vi "Detect Objects with YOLOV3-tiny.vi"() -> ()   [LabVIEW 2020, in "examples.lvlib"]
uses:
  examples.lvlib
  feature_detection/DNN Detection Model/Detection.ctl
  feature_detection/DNN Detection Model/Rectangle Corners.ctl
  common/Image Point (Integer).ctl
  feature_detection/DNN Detection Model/Model Parameters.ctl
  common/Image Size (Integer).ctl
  common/Object Point (Float).ctl
  <vilib>/Utility/sysdir.llb/System Directory Type.ctl
  feature_detection/DNN Detection Model/DNN Detection Model.lvclass/DNN Detection Model.ctl
  image/ARGB Colour.ctl
  image/New Image (ARGB Preallocated).vi
  image/Copy Pixmap to Image (ARGB Flatten Mask).vi
  feature_detection/DNN Detection Model/Detect (ARGB).vi
  image/Draw Rectangle (ARGB).vi
  image/Draw Text (ARGB).vi
  image/Draw Image to Picture (ARGB).vi
  image/New Image (ARGB Preallocated).vi/3321fa97-f432-4e1e-8db9-a0df79aed21b.vi
  image/ARGB Colour to U32 Pixel Value.vi
  image/Copy Pixmap to Image (ARGB Flatten Mask).vi/7d03ccf7-b889-4e8d-9f2a-57831e73dbde.vi
  feature_detection/DNN Detection Model/Detect (ARGB).vi/e837249a-f575-44a9-ab73-66ed6d7d79a4.vi
  image/Draw Rectangle (ARGB).vi/7e6fb015-3761-4366-a0a7-e436eb229083.vi
  image/Draw Text (ARGB).vi/0015c4fc-6a12-4f82-815b-6c2f827f408b.vi
  image/Draw Image to Picture (ARGB).vi/8cd07b1b-062e-4fe4-9e87-2eb3dc89fe0e.vi
  image/FixPixmap.vi
  image/Default8bitColourMap.vi
  <vilib>/Utility/file.llb/Read Delimited Spreadsheet (string).vi
  feature_detection/DNN Detection Model/Create (Darknet).vi
  <vilib>/Utility/error.llb/Error Cluster From Error Code.vi
  feature_detection/DNN Detection Model/DNN Detection Model.lvclass
  common/common.lvlib
  image/image.lvlib
  <vilib>/picture/picture.llb/imagedata.ctl
panel:
  out "Picture":picture
  out "Detections":T1[](array[typedef])
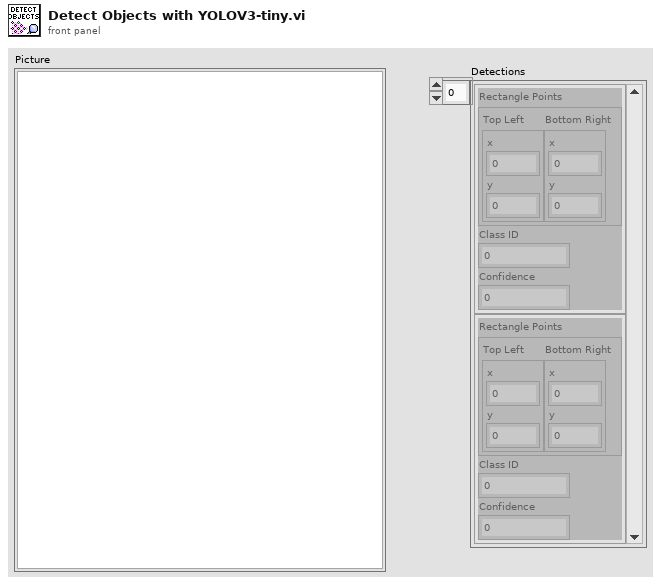
[diagram p1: front panel]
types:
  T1 = typedef "feature_detection.lvlib/DNN Detection Model.lvclass/Detection.ctl" = cluster{"Rectangle Points":T2, "Class ID":i32, "Confidence":sgl}
  T2 = typedef "feature_detection.lvlib/DNN Detection Model.lvclass/Rectangle Corners.ctl" = cluster{"Top Left":T3, "Bottom Right":T3}
  T3 = typedef "common.lvlib/Image Point (Integer).ctl" = cluster{"x":i32, "y":i32}
  T4 = typedef "feature_detection.lvlib/DNN Detection Model.lvclass/Model Parameters.ctl" = cluster{"Image Size":T5, "Mean":T6, "Scale":dbl, "Expects RGB Channel Order":bool, "Crop":bool}
  T5 = typedef "common.lvlib/Image Size (Integer).ctl" = cluster{"Width":u16, "Height":u16}
  T6 = typedef "common.lvlib/Object Point (Float).ctl" = cluster{"x":dbl, "y":dbl, "z":dbl}
  T7 = typedef "System Directory Type.ctl" = i32
  T8 = typedef "imagedata.ctl" = cluster{"image type":i32, "image depth":i32, "image":u8[], "mask":u8[], "colors":u32[], "Rectangle":cluster{"left":i16, "top":i16, "right":i16, "bottom":i16}}
  T9 = typedef "image.lvlib/ARGB Image.ctl" = refnum<data-value>
  T10 = typedef "image.lvlib/ARGB Colour.ctl" = cluster{"Alpha":u8, "RGB":u32}
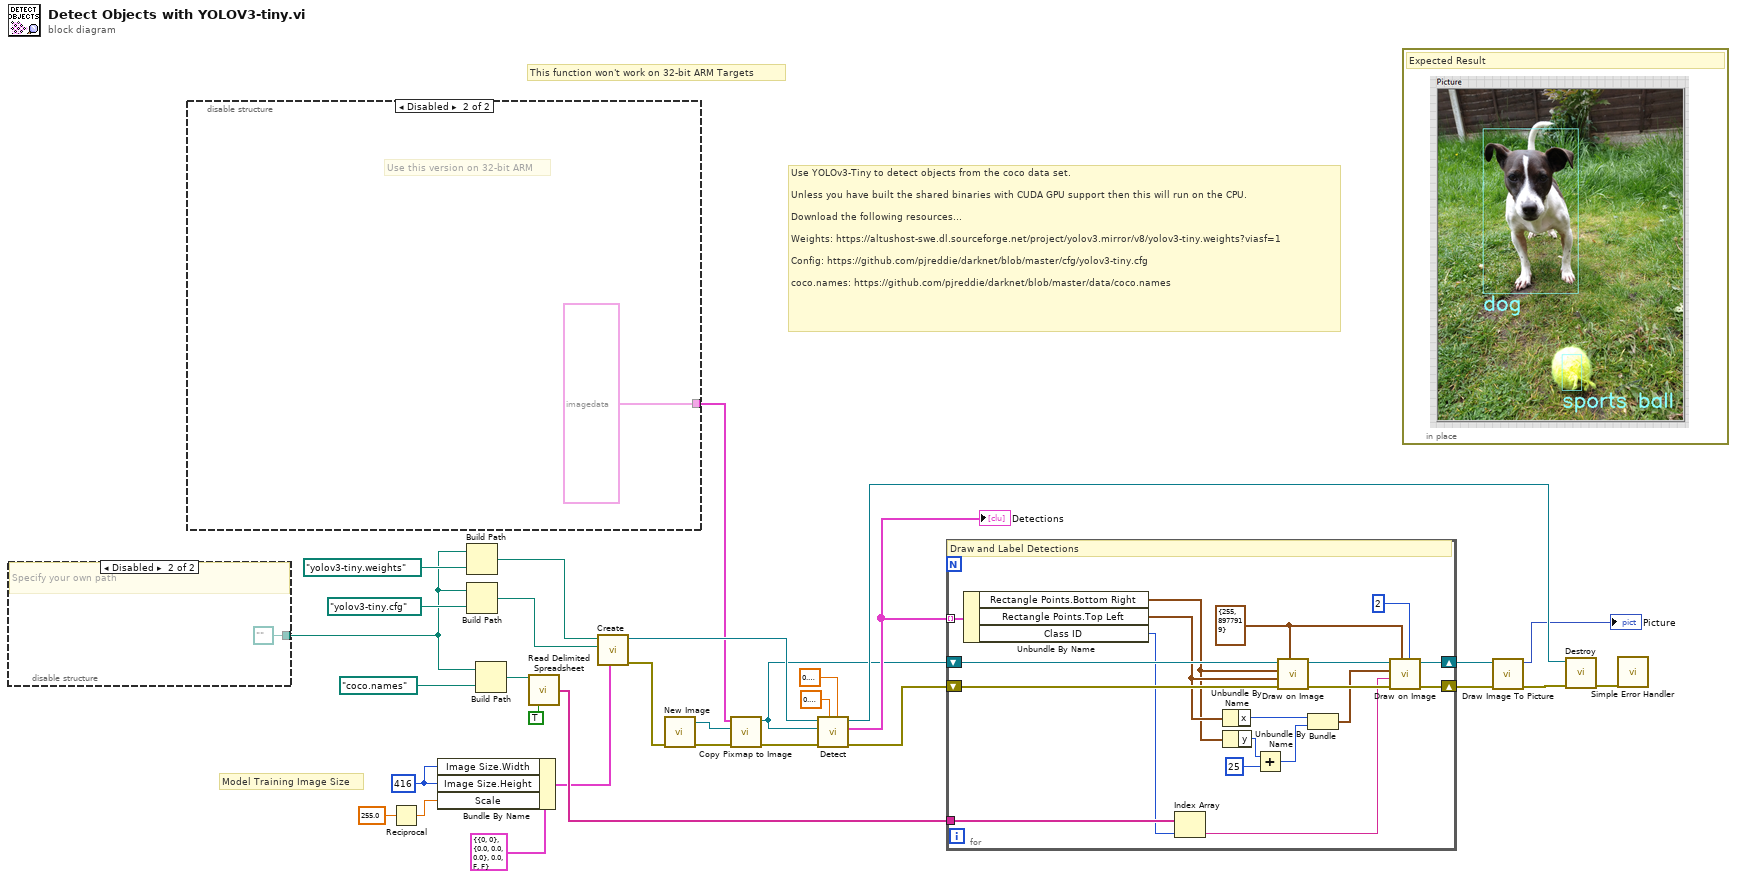
[diagram p0: block diagram]
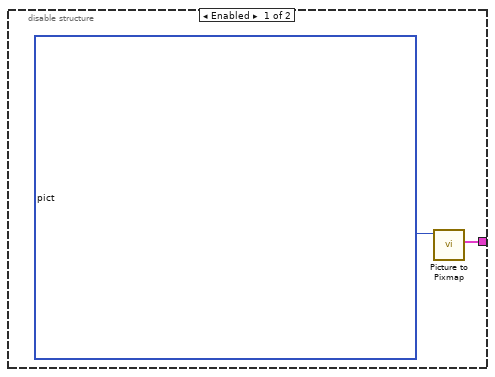
[diagram p2: hidden frame]
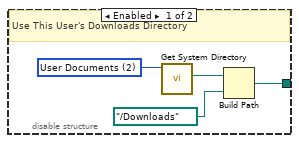
[diagram p3: hidden frame]
diagram:
  w19 = u16 416 ("Image Size.Width")
  # "This function won't work on 32-bit ARM Targets"
  # "Model Training Image Size"
  # "Use YOLOv3-Tiny to detect objects from the coco data set.\n\nUnless you have built the shared binaries with CUDA GPU support then this will run on the CPU.\n\nDownload the following resources...\n\nWeights: https://altushost-swe.dl.sourceforge.net/project/yolov3.mirror/v8/yolov3-tiny.weights?viasf=1\n\nConfig: https://github.com/pjreddie/darknet/blob/master/cfg/yolov3-tiny.cfg\n\ncoco.names: https://github.com/pjreddie/darknet/blob/master/data/coco.names"
  n1 = disable-structure shown="Disabled" {
    disable-tunnel: [w32 path "" ("appended path")] -> w16
    frame Enabled {
      w35 = T7 2 items=["User Home"=0, "User Desktop"=1, "User Documents"=2, "User Application Data"=3, "User Preferences"=4, "User Temporary"=5, "Public Documents"=6, "Public Application Data"=7, "Public Preferences"=8, "Public Cache"=13, "System Core Libraries"=9, "System Installed Libraries"=10, "Application Files"=11, "Boot Volume Root"=12] ("system directory type")
      # "Use This User's Downloads Directory"
      n2 = call <vilib>:"Get System Directory.vi"("system directory type"=w35) -> ("system directory"=w34:path)  [unwired: 10 in]
      n3 = Build Path(base path=w34, name or relative path=path "../Downloads") -> (appended path=w32:path)
    }
    frame Disabled {
      # "Specify your own path"
    }
  }
  n4 = disable-structure shown="Disabled" {
    disable-tunnel: [w37 T8 {"image type"=0, "image depth"=24, "image"=array[562500 elements], "mask"=[], "colors"=[], "Rectangle"={"left"=0, "top"=0, "right"=375, "bottom"=500}} ("image data")] -> w6
    frame Enabled {
      n5 = call <vilib>:"Picture to Pixmap.vi"("picture"=picture bytes[562530] ("Picture")) -> ("image data"=w37:T8)  [unwired: 9 in, 1 out]
    }
    frame Disabled {
      # "Use this version on 32-bit ARM"
    }
  }
  n6 = Reciprocal(x=255.0) -> (1/x=w20:dbl)
  n7 = Bundle By Name(cluster=T4 {"Image Size"={"Width"=0, "Height"=0}, "Mean"={"x"=0.0, "y"=0.0, "z"=0.0}, "Scale"=0.0, "Expects RGB Channel Order"=FALSE, "Crop"=FALSE} ("Image Handling Properties"), "Image Size.Width"=w19, "Image Size.Height"=w19, "Scale"=w20) -> (w21:T4)
  n8 = Build Path(base path=w16, name or relative path=path "yolov3-tiny.weights") -> (appended path=w26:path)
  n9 = Build Path(base path=w16, name or relative path=path "yolov3-tiny.cfg") -> (appended path=w23:path)
  n10 = Build Path(base path=w16, name or relative path=path "coco.names") -> (appended path=w13:path)
  n11 = call-poly <vilib>:"Read Delimited Spreadsheet.vi"("file path (dialog if empty)"=w13, "transpose? (F)"=TRUE) -> ("first row"=w31:string[])  [unwired: 8 in, 5 out]
  n12 = call-poly "Create.vi"("Image Handling Properties"=w21, "Config (*.cfg)"=w23, "Darknet Weights (*.weights)"=w26) -> ("error out"=w30:errorcluster, "DNN Detection Model"=w28:refnum<class "DNN Detection Model.lvclass">)  [unwired: 7 in]
  n13 = call-poly "New Image.vi"("error in (no error)"=w30) -> ("error out"=w2:errorcluster, "ARGB Image"=w1:T9)  [unwired: 9 in]
  n14 = call-poly "Copy Pixmap to Image.vi"("error in (no error)"=w2, "ARGB Image Destination in"=w1, "Pixmap Image Data"=w6) -> ("error out"=w4:errorcluster, "ARGB Image Destination"=w3:T9)  [unwired: 7 in]
  n15 = call-poly "Detect.vi"("Non-Maxium Suppression Threshold"=sgl 0.1, "Confidence Threshold"=sgl 0.2, "error in (no error)"=w4, "ARGB Image in"=w3, "DNN Detection Model in"=w28) -> ("error out"=w12:errorcluster, "Detections"=w11:T1[], "DNN Detection Model"=w29:refnum<class "DNN Detection Model.lvclass">)  [unwired: 4 in]
  "Detections" <- w11
  n16 = for {
    tunnel: w11 -> [w58] mode=indexing
    shift-right: [w53] -> w9
    shift-left: w12 -> [w57]
    shift-right: [w52] -> w10
    shift-left: w3 -> [w56]
    tunnel: w31 -> [w55]
    w50 = T10 {"Alpha"=255, "RGB"=8977919} ("ARGB Colour")
    # "Draw and Label Detections"
    n17 = Unbundle By Name(w58) -> ("Rectangle Points.Bottom Right"=w45:T3, "Rectangle Points.Top Left"=w46:T3, "Class ID"=w47:i32)
    n18 = Index Array(array=w55, index=w47) -> (element=w49:string)
    n19 = Unbundle By Name(w46) -> ("x"=w44:i32)
    n20 = Unbundle By Name(w45) -> ("y"=w43:i32)
    n21 = Add(x=w43, y=25) -> (x+y=w41:i32)
    n22 = call-poly "Draw on Image.vi"("ARGB Colour"=w50, "error in (no error)"=w57, "Point B"=w46, "Point A"=w45, "ARGB Image in"=w56) -> ("error out"=w54:errorcluster, "ARGB Image"=w51:T9)  [unwired: 5 in]
    n23 = Bundle("x"=w44, w41) -> (w42:cluster{"x":i32, i32})  [unwired: 1 in]
    n24 = call-poly "Draw on Image.vi"("Thickness (Default: 1)"=2, "ARGB Colour"=w50, "error in (no error)"=w54, "Text"=w49, "Origin"=w42, "ARGB Image in"=w51) -> ("error out"=w53:errorcluster, "ARGB Image"=w52:T9)  [unwired: 4 in]
  }
  n25 = in-place {
    # "Expected Result"
  }
  n26 = call-poly "Draw Image To Picture.vi"("error in (no error)"=w9, "ARGB Image Source in"=w10) -> ("error out"=w8:errorcluster, "Picture"=→"Picture":picture)  [unwired: 8 in]
  n27 = call "Destroy.vi"("error in (no error)"=w8, "DNN Detection Model"=w29) -> ("error out"=w5:errorcluster)  [unwired: 9 in]
  n28 = call <vilib>:"Simple Error Handler.vi"("error in (no error)"=w5) -> ()  [unwired: 4 in, 5 out]
